vi "Read As Stream_WaitForCompletion.vi"(6 "millisecondsTimeout (-1 indefinite)":i32=-1, 7 "CloseDestinationStream [T]":bool=TRUE, 8 "error in (no error)":errorcluster, 11 "HttpContent in":refnum<class "HttpContent.lvclass">) -> (0 "error out":errorcluster, 1 "IsCompleted":bool, 3 "HttpContent out":refnum<class "HttpContent.lvclass">, 4 "Canceled":bool)   [LabVIEW 2018, in "LabVIEWHTTPClient_NET.lvlib" / "HttpContent.lvclass"]
uses:
  HttpContent.lvclass
  HttpContent.lvclass/HttpContent.ctl
  Types/HttpNet_error_enum.ctl
  Accessors/Read NET_StreamTask.vi
  LabVIEWHTTPClient_NET/LabVIEWHTTPClient_NET.lvlib
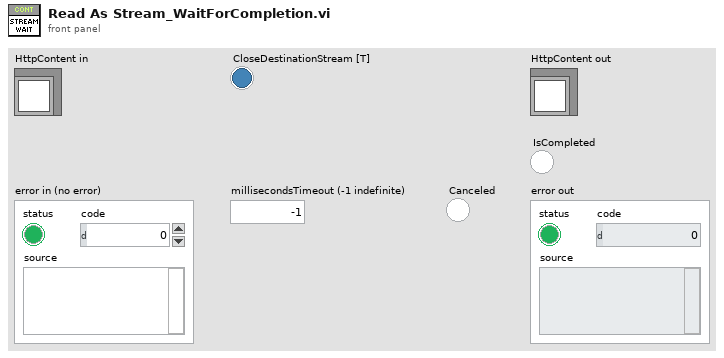
[diagram p1: front panel]
types:
  T1 = typedef "LabVIEWHTTPClient_NET.lvlib/HttpNet_error_enum.ctl" = enum16{"REST method is not available", "URL cannot be blank", "Output filepath cannot be empty", "Input filepath cannot be empty", "Internal .NET error %s", "Output filepath cannot be directory", "Download Task no longer exists", "Mutipart Put not supported from REST Client Interface.  Please revert to lower level classes"}
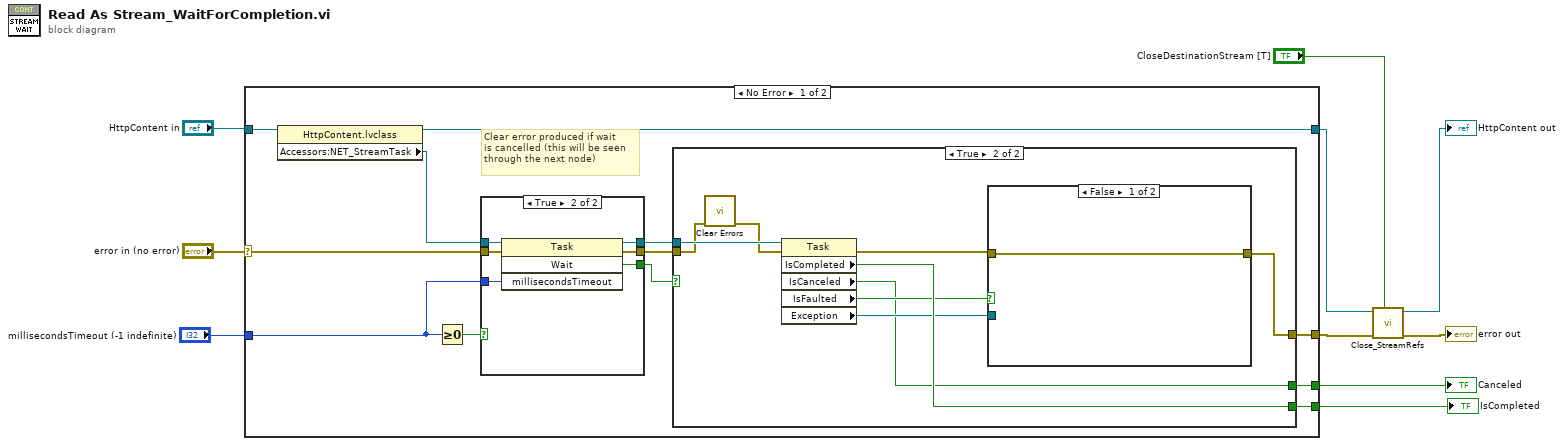
[diagram p0: block diagram]
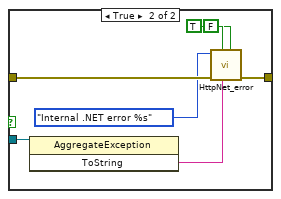
[diagram p3: hidden frame]
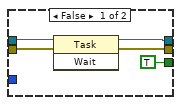
[diagram p4: hidden frame]
diagram:
  n1 = case shown="No Error" "error in (no error)" {
    selector: "error in (no error)" -> [w22 w53]
    tunnel: [w14 _] -> w9
    tunnel: [w20 _] -> w8
    tunnel: "HttpContent in" -> [w19 w52]
    tunnel: [w18 w53] -> w4
    tunnel: [w16 w52] -> w6
    tunnel: "millisecondsTimeout (-1 indefinite)" -> [w13 _]
    frame No Error {
      # "Clear error produced if wait\nis cancelled (this will be seen \nthrough the next node)"
      n2 = property class="HttpContent.lvclass"(reference=w19) -> (reference out=w16:refnum<class "HttpContent.lvclass">, "Accessors:NET_StreamTask"=w15:refnum<k24>)  [unwired: 1 in, 1 out]
      n3 = Greater Or Equal To 0?(x=w13) -> (x >= 0?=w12:bool)
      n4 = case shown="True" w12 {
        tunnel: w22 -> [w43 w51]
        tunnel: [w45 w50] -> w21
        tunnel: [w42 w49] -> w17
        tunnel: w15 -> [w44 w48]
        tunnel: w13 -> [_ w47]
        tunnel: [TRUE ("Wait") w46] -> w11
        frame False {
          n5 = invoke class="Task" method="Wait"(reference=w44, error in=w43) -> (reference out=w45:refnum<k24>, error out=w42:errorcluster)  [unwired: 1 in, 1 out]
        }
        frame True {
          n6 = invoke class="Task" method="Wait"(reference=w48, error in=w51, "millisecondsTimeout"=w47) -> (reference out=w50:refnum<k24>, error out=w49:errorcluster, "Wait"=w46:bool)  [unwired: 1 in, 1 out]
        }
      }
      n7 = case shown="True" w11 {
        tunnel: w21 -> [_ w32]
        tunnel: [_ w30] -> w20
        tunnel: [w23 w27] -> w18
        tunnel: w17 -> [w23 w26]
        tunnel: [_ w24] -> w14
        frame False {
        }
        frame True {
          n8 = call <vilib>:"Clear Errors.vi"("error in (no error)"=w26) -> ("error out"=w25:errorcluster)  [unwired: 5 in, 1 out]
          n9 = property class="Task"(reference=w32, error in=w25) -> (error out=w31:errorcluster, "IsCompleted"=w30:bool, "IsCanceled"=w24:bool, "IsFaulted"=w29:bool, "Exception"=w28:refnum<k24>)  [unwired: 1 out]
          n10 = case shown="False" w29 {
            tunnel: w28 -> [_ w40]
            tunnel: w31 -> [w33 w39]
            tunnel: [w33 w34] -> w27
            frame False {
            }
            frame True {
              n11 = invoke class="AggregateException" method="ToString"(reference=w40) -> ("ToString"=w38:string)  [unwired: 2 in, 2 out]
              n12 = call "HttpNet_error.vi"("ShowCallChain [T]"=FALSE, "IncludedString"=w38, "OverrideExistingErrors [T]"=TRUE, "Error In"=w39, "Error"=HttpNet_error_enum."Internal .NET error %s") -> ("Error Out"=w34:errorcluster)  [unwired: 6 in]
            }
          }
        }
      }
    }
    frame Error {
    }
  }
  "Canceled" <- w9
  "IsCompleted" <- w8
  n13 = call "Close_StreamRefs.vi"("CloseDestinationStream [T]"="CloseDestinationStream [T]", "error in (no error)"=w4, "HttpContent in"=w6) -> ("error out"=→"error out":errorcluster, "HttpContent out"=→"HttpContent out":refnum<class "HttpContent.lvclass">)  [unwired: 7 in]
